vi "New NIErrLog Log Provider.vi"(7 "context":string, 8 "error in (no error)":errorcluster, 10 "level":T1 items=["OFF"=0, "FATAL"=100, "ERROR"=200, "WARN"=300, "INFO"=400, "DEBUG"=500, "TRACE"=600, "ALL"=65535]) -> (0 "error out":errorcluster, 3 "Queue Log Provider":refnum<data-value>)   [LabVIEW 2019, in "LVCOOOP.lvlib" / "Utility API.lvlib" / "NIErrLog Log Provider.lvclass"]
uses:
  NIErrLog Log Provider.lvclass
  Log Service/public/level.ctl
  NIErrLog Log Provider.lvclass/NIErrLog Log Provider.ctl
  Log Service/Log Service.lvclass
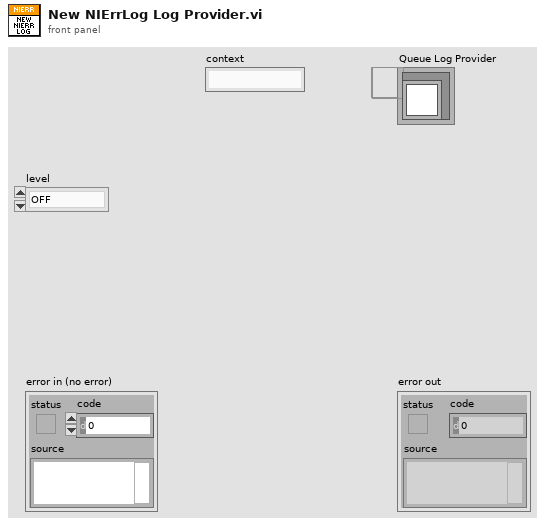
[diagram p1: front panel]
types:
  T1 = typedef "LVCOOOP.lvlib/Utility API.lvlib/Log Service.lvclass/level.ctl" = u16
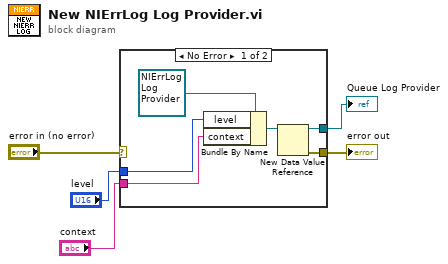
[diagram p0: block diagram]
diagram:
  n1 = case shown="No Error" "error in (no error)" {
    selector: "error in (no error)" -> [_ w12]
    tunnel: [w9 w12] -> w4
    tunnel: [w7 _] -> w3
    tunnel: "context" -> [w11 _]
    tunnel: "level" -> [w10 _]
    frame No Error {
      n2 = Bundle By Name(cluster=refnum<class "NIErrLog Log Provider.lvclass"> refnum ("Queue Log Provider in"), "level"=w10, "context"=w11) -> (w8:refnum<class "NIErrLog Log Provider.lvclass">)
      n3 = New Data Value Reference(data value=w8) -> (data value reference=w7:refnum<data-value>, error out=w9:errorcluster)  [unwired: 1 in]
    }
    frame Error {
    }
  }
  "error out" <- w4
  "Queue Log Provider" <- w3
